vi "SendDrivingCAN.vi"(11 "CANTXQueueIn":T1) -> (3 "CANTXQueueOut":T1)   [LabVIEW 2015]
uses:
  CAN/TX Library/CAN Message Queue.ctl
  CAN/TX Library/CAN Message.ctl
  <vilib>/RioEmbeddedCAN/RioEmbeddedCAN.llb/CANFrameControl.ctl
  Global Data.vi
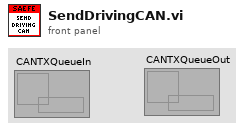
[diagram p1: front panel]
types:
  T1 = typedef "CAN Message Queue.ctl" = refnum<k33>
  T2 = typedef "CANFrameControl.ctl" = cluster{"identifier":u32, "extended?":bool, "type":u8, "payload":u8[]}
  T3 = typedef "Lap Statistics.ctl" = cluster{"rBrakeBalLast":dbl}
  T4 = typedef "MC Temp 2.ctl" = cluster{"TMCControlBoard":dbl, "TMCRTD1":dbl, "TMCRTD2":dbl, "TMCRTD3":dbl}
  T5 = typedef "BMS Telemetry.ctl" = cluster{"bBMSIgnition":bool, "bBMSChargerMains":bool, "bBMSFastCharge":bool, "bBMSChargerEnabled":bool, "eBMSCarState":enum16{"Off", "On, Not Charging", "Charging", "Charging Finished", "Charging Error"}, "eBMSChargingState":enum16{"Disconnected", "Pre-charging", "Main Charging", "Balancing", "Charging Finished OK", "Charging Error"}, "tBMSChargeStage":u16, "eBMSLastChargeError":enum16{"No Error", "No Cell Communication", "No Cell Communication - Non CAN Charger", "Maximum charging stage duration expired", "Cell Communication Lost during Charge", "Cannot set balancing voltage", "Cell temps too high", "No Comms so can't determine temp", "# of Cells Mismatch", "Cells Overvoltage", "Cell Protection Event occured."}, "NBMSNumCells":u8, "bBMSUnderVProtection":bool, "bBMSOverVProtection":bool, "bBMSOverTProtection":bool, "bBMSLeakageProtection":bool, "bBMSNoCellCommsError":bool, "bBMSLowVReduction":bool, "bBMSHighTReduction":bool, "VCellMin":dbl, "VCellMax":dbl, "VCellMean":dbl, "VTotal":dbl, "TCellMin":dbl, "TCellMax":dbl, "TCellMean":dbl, "VCells":cluster{"[51]":dbl, "[53]":dbl, "[54]":dbl, "[55]":dbl, "[56]":dbl, "[57]":dbl, "[58]":dbl, "[59]":dbl, "[60]":dbl, "[61]":dbl, "[62]":dbl, "[63]":dbl, "[64]":dbl, "[65]":dbl, "[66]":dbl, "[67]":dbl, "[34]":dbl, "[35]":dbl, "[36]":dbl, "[37]":dbl, "[38]":dbl, "[39]":dbl, "[40]":dbl, "[41]":dbl, "[42]":dbl, "[43]":dbl, "[44]":dbl, "[45]":dbl, "[46]":dbl, "[47]":dbl, "[48]":dbl, "[49]":dbl, "[50]":dbl, "[17]":dbl, "[18]":dbl, "[19]":dbl, "[20]":dbl, "[21]":dbl, "[22]":dbl, "[23]":dbl, "[24]":dbl, "[25]":dbl, "[26]":dbl, "[27]":dbl, "[28]":dbl, "[29]":dbl, "[30]":dbl, "[31]":dbl, "[32]":dbl, "[33]":dbl, "[0]":dbl, "[1]":dbl, "[2]":dbl, "[3]":dbl, "[4]":dbl, "[5]":dbl, "[6]":dbl, "[7]":dbl, "[8]":dbl, "[9]":dbl, "[10]":dbl, "[11]":dbl, "[12]":dbl, "[13]":dbl, "[14]":dbl, "[15]":dbl, "[16]":dbl, "[52] 2":dbl}, "TBMSCells":cluster{"[55]":dbl, "[56]":dbl, "[57]":dbl, "[58]":dbl, "[59]":dbl, "[60]":dbl, "[61]":dbl, "[62]":dbl, "[63]":dbl, "[64]":dbl, "[65]":dbl, "[66]":dbl, "[67]":dbl, "[68]":dbl, "[69]":dbl, "[70]":dbl, "[17]":dbl, "[38]":dbl, "[39]":dbl, "[40]":dbl, "[41]":dbl, "[42]":dbl, "[43]":dbl, "[44]":dbl, "[45]":dbl, "[46]":dbl, "[47]":dbl, "[48]":dbl, "[49]":dbl, "[50]":dbl, "[51]":dbl, "[52]":dbl, "[53]":dbl, "[54]":dbl, "[21]":dbl, "[22]":dbl, "[23]":dbl, "[24]":dbl, "[25]":dbl, "[26]":dbl, "[27]":dbl, "[28]":dbl, "[29]":dbl, "[30]":dbl, "[31]":dbl, "[32]":dbl, "[33]":dbl, "[34]":dbl, "[35]":dbl, "[36]":dbl, "[37]":dbl, "[0]":dbl, "[1]":dbl, "[2]":dbl, "[3]":dbl, "[4]":dbl, "[5]":dbl, "[6]":dbl, "[7]":dbl, "[8]":dbl, "[9]":dbl, "[10]":dbl, "[11]":dbl, "[12]":dbl, "[13]":dbl, "[14]":dbl, "[15]":dbl, "[16]":dbl}, "bChargerConnected":bool, "VChargerSetpoint":dbl, "IChargerSetpoint":dbl, "VChargerActual":dbl, "IChargerActual":dbl, "BCells":cluster{"[51]":dbl, "[52]":dbl, "[53]":dbl, "[54]":dbl, "[55]":dbl, "[56]":dbl, "[57]":dbl, "[58]":dbl, "[59]":dbl, "[60]":dbl, "[61]":dbl, "[62]":dbl, "[63]":dbl, "[64]":dbl, "[65]":dbl, "[66]":dbl, "[67]":dbl, "[34]":dbl, "[35]":dbl, "[36]":dbl, "[37]":dbl, "[38]":dbl, "[39]":dbl, "[40]":dbl, "[41]":dbl, "[42]":dbl, "[43]":dbl, "[44]":dbl, "[45]":dbl, "[46]":dbl, "[47]":dbl, "[48]":dbl, "[49]":dbl, "[50]":dbl, "[17]":dbl, "[18]":dbl, "[19]":dbl, "[20]":dbl, "[21]":dbl, "[22]":dbl, "[23]":dbl, "[24]":dbl, "[25]":dbl, "[26]":dbl, "[27]":dbl, "[28]":dbl, "[29]":dbl, "[30]":dbl, "[31]":dbl, "[32]":dbl, "[33]":dbl, "[0]":dbl, "[1]":dbl, "[2]":dbl, "[3]":dbl, "[4]":dbl, "[5]":dbl, "[6]":dbl, "[7]":dbl, "[8]":dbl, "[9]":dbl, "[10]":dbl, "[11]":dbl, "[12]":dbl, "[13]":dbl, "[14]":dbl, "[15]":dbl, "[16]":dbl}, "bNewVCellMinSample":bool, "Battery Temp":cluster{"[0]":dbl, "[1]":dbl, "[2]":dbl, "[3]":dbl, "[4]":dbl, "[5]":dbl, "[6]":dbl, "[7]":dbl, "[8]":dbl, "[9]":dbl, "[10]":dbl, "[11]":dbl, "[12]":dbl, "[13]":dbl, "[14]":dbl, "[15]":dbl, "[16]":dbl, "[17]":dbl, "[18]":dbl, "[19]":dbl, "[20]":dbl, "[21]":dbl, "[22]":dbl, "[23]":dbl, "[24]":dbl, "[25]":dbl, "[26]":dbl, "[27]":dbl, "[28]":dbl, "[29]":dbl, "[30]":dbl, "[31]":dbl, "[32]":dbl, "[33]":dbl, "[34]":dbl, "[35]":dbl, "[36]":dbl, "[37]":dbl, "[38]":dbl, "[39]":dbl, "[40]":dbl, "[41]":dbl, "[42]":dbl, "[43]":dbl, "[44]":dbl, "[45]":dbl, "[46]":dbl, "[47]":dbl, "[48]":dbl, "[49]":dbl, "[50]":dbl, "[51]":dbl, "[52]":dbl, "[53]":dbl, "[54]":dbl, "[55]":dbl, "[56]":dbl, "[57]":dbl, "[58]":dbl, "[59]":dbl, "[60]":dbl, "[61]":dbl, "[62]":dbl, "[63]":dbl, "[64]":dbl, "[65]":dbl, "[66]":dbl, "[67]":dbl, "[68]":dbl, "[69]":dbl, "[71]":dbl, "[70]":dbl, "[0] 2":dbl, "[1] 2":dbl, "[2] 2":dbl, "[3] 2":dbl, "[4] 2":dbl, "[5] 2":dbl, "[6] 2":dbl, "[7] 2":dbl, "[8] 2":dbl, "[9] 2":dbl, "[10] 2":dbl, "[11] 2":dbl, "[12] 2":dbl, "[13] 2":dbl, "[14] 2":dbl, "[15] 2":dbl, "[16] 2":dbl, "[17] 2":dbl, "[18] 2":dbl, "[19] 2":dbl, "[20] 2":dbl, "[21] 2":dbl, "[22] 2":dbl, "[23] 2":dbl, "[24] 2":dbl, "[25] 2":dbl, "[26] 2":dbl, "[27] 2":dbl, "[28] 2":dbl, "[29] 2":dbl, "[30] 2":dbl, "[31] 2":dbl, "[32] 2":dbl, "[33] 2":dbl, "[34] 2":dbl, "[35] 2":dbl, "[36] 2":dbl, "[37] 2":dbl, "[38] 2":dbl, "[39] 2":dbl, "[40] 2":dbl, "[41] 2":dbl, "[42] 2":dbl, "[43] 2":dbl, "[44] 2":dbl, "[45] 2":dbl, "[46] 2":dbl, "[47] 2":dbl, "[48] 2":dbl, "[49] 2":dbl, "[50] 2":dbl, "[51] 2":dbl, "[52] 3":dbl, "[53] 2":dbl, "[54] 2":dbl, "[55] 2":dbl, "[56] 2":dbl, "[57] 2":dbl, "[58] 2":dbl, "[59] 2":dbl, "[60] 2":dbl, "[61] 2":dbl, "[62] 2":dbl, "[63] 2":dbl, "[64] 2":dbl, "[65] 2":dbl, "[66] 2":dbl, "[67] 2":dbl, "[68]2":dbl, "[69]2":dbl, "[70]2":dbl, "[71]2":dbl, "[0] 3":dbl, "[1] 3":dbl, "[2] 3":dbl, "[3] 3":dbl, "[4] 3":dbl, "[5] 3":dbl, "[6] 3":dbl, "[7] 3":dbl, "[8] 3":dbl, "[9] 3":dbl, "[10] 3":dbl, "[11] 3":dbl, "[12] 3":dbl, "[13] 3":dbl, "[14] 3":dbl, "[15] 3":dbl, "[16] 3":dbl, "[17] 3":dbl, "[18] 3":dbl, "[19] 3":dbl, "[20] 3":dbl, "[21] 3":dbl, "[22] 3":dbl, "[23] 3":dbl, "[24] 3":dbl, "[25] 3":dbl, "[26] 3":dbl, "[27] 3":dbl, "[28] 3":dbl, "[29] 3":dbl, "[30] 3":dbl, "[31] 3":dbl, "[32] 3":dbl, "[33] 3":dbl, "[34] 3":dbl, "[35] 3":dbl, "[36] 3":dbl, "[37] 3":dbl, "[38] 3":dbl, "[39] 3":dbl, "[40] 3":dbl, "[41] 3":dbl, "[42] 3":dbl, "[43] 3":dbl, "[44] 3":dbl, "[45] 3":dbl, "[46] 3":dbl, "[47] 3":dbl, "[48] 3":dbl, "[49] 3":dbl, "[50] 3":dbl, "[51] 3":dbl, "[52] 4":dbl, "[53] 3":dbl, "[54] 3":dbl, "[55] 3":dbl, "[56] 3":dbl, "[57] 3":dbl, "[58] 3":dbl, "[59] 3":dbl, "[60] 3":dbl, "[61] 3":dbl, "[62] 3":dbl, "[63] 3":dbl, "[64] 3":dbl, "[65] 3":dbl, "[66] 3":dbl, "[67] 3":dbl, "[68]3":dbl, "[69]3":dbl, "[70]3":dbl, "[71]3":dbl, "[4] 4":dbl, "[5] 4":dbl, "[6] 4":dbl, "[7] 4":dbl, "[8] 4":dbl, "[9] 4":dbl, "[10] 4":dbl, "[11] 4":dbl, "[12] 4":dbl, "[13] 4":dbl, "[14] 4":dbl, "[15] 4":dbl, "[16] 4":dbl, "[17] 4":dbl, "[18] 4":dbl, "[19] 4":dbl, "[20] 4":dbl, "[21] 4":dbl, "[22] 4":dbl, "[23] 4":dbl, "[24] 4":dbl, "[25] 4":dbl, "[26] 4":dbl, "[27] 4":dbl, "[28] 4":dbl, "[29] 4":dbl, "[30] 4":dbl, "[31] 4":dbl, "[32] 4":dbl, "[33] 4":dbl, "[17] 9":dbl, "[0] 9":dbl, "[51] 8":dbl, "[34] 8":dbl, "[17] 8":dbl, "[0] 8":dbl, "[34] 4":dbl, "[35] 4":dbl, "[36] 4":dbl, "[37] 4":dbl, "[38] 4":dbl, "[39] 4":dbl, "[40] 4":dbl, "[41] 4":dbl, "[42] 4":dbl, "[43] 4":dbl, "[44] 4":dbl, "[45] 4":dbl, "[46] 4":dbl, "[47] 4":dbl, "[48] 4":dbl, "[49] 4":dbl, "[50] 4":dbl, "[34] 9":dbl, "[51] 4":dbl, "[52] 5":dbl, "[53] 4":dbl, "[54] 4":dbl, "[55] 4":dbl, "[56] 4":dbl, "[57] 4":dbl, "[58] 4":dbl, "[59] 4":dbl, "[60] 4":dbl, "[61] 4":dbl, "[62] 4":dbl, "[63] 4":dbl, "[64] 4":dbl, "[65] 4":dbl, "[66] 4":dbl, "[67] 4":dbl, "[51] 9":dbl}, "TBMSMax":dbl, "TBMSMin":dbl, "TBMSMean":dbl}
  T6 = typedef "MC Temp 1.ctl" = cluster{"TMCModuleA":dbl, "TMCModuleB":dbl, "TMCModuleC":dbl, "TMCGateDriver":dbl}
  T7 = typedef "MC Temp 3.ctl" = cluster{"TMCRTD4":dbl, "TMCRTD5":dbl, "TMotor":dbl, "MTorqueShudder":dbl}
  T8 = typedef "FPGA Telemetry.ctl" = cluster{"CPU Load":cluster{"Total (%)":dbl, "Time Critical (%)":dbl, "Timed Structures (%)":dbl, "High (%)":dbl, "Above Normal (%)":dbl, "Normal (%)":dbl, "Background (%)":dbl, "Idle (%)":dbl, "ISR (%)":dbl}, "SVehicleStatus":cluster{"BMS Status":T9, "MC Status":T9, "Shutdown Status":T9, "sbRIO Status":T9, "Vehicle Status":T9, "Shutdown State":enum16{"NI.SC.Initial", "NI.SC.History", "NI.SC.ShallowHistory", "NI.SC.Terminal", "Coolant Pump Started/AIR's On", "AIRs On", "Precharge", "TSMS Off"}, "AIR Status":T12, "Remote Return to Pits":bool, "Reason for Shutdown":T13, "MC State Machine Status":enum16{"NI.SC.Initial", "NI.SC.History", "NI.SC.ShallowHistory", "NI.SC.Terminal", "Broadcast Diag", "Let Current Drop then Disable AIR's", "Enabled", "Disabled"}}, "iPhone HF Data":cluster{"gXiPhone":dbl, "gYiPhone":dbl, "gZiPhone":dbl, "nYawXiPhone":dbl, "nYawYiPhone":dbl, "nYawZiPhone":dbl}, "iPhone LF Data":cluster{"nLatiPhone":dbl, "nLongiPhone":dbl, "nGPSiPhone":dbl}, "stop":bool, "VSupplyOffset":fxp<+,12,4>, "VsbRIOSupply":fxp<+/-,25,6>, "bFPGALED":bool, "TSBRIO":fxp<+/-,33,17>, "rTPS2Unscaled":fxp<+/-,16,1>, "rTPS1Unscaled":fxp<+/-,16,1>, "bTPSConsistent":bool, "bTPSInRange":bool, "rThrottle":fxp<+/-,33,22>, "VTPS2":fxp<+/-,24,5>, "rTPS2":fxp<+/-,31,22>, "VTPS1":fxp<+/-,24,5>, "rTPS1":fxp<+/-,31,22>, "rTPS2Max":fxp<+,16,4>, "rTPS2Min":fxp<+,16,4>, "rTPS1Max":fxp<+,16,4>, "rTPS1Min":fxp<+,16,4>, "bCoolantPumpEnable":bool, "bRTDSEnable":bool, "bTSMSInStatus":bool, "bPosAIREnable":bool, "bBMSOK":bool, "bIMDOK":bool, "bBSPDOK":bool, "bSBRIOOK2":bool, "bSBRIOOK1":bool, "bTSMSOutStatus":bool, "eGreenDash":T14, "eYellowDash":T14, "eRedDash":T14, "bMotorControllerEnable":bool, "tCurrentLap":u32, "bNewLap":bool, "tLastLap":u32, "tLapMin":u32, "V5VSupply":fxp<+/-,24,5>, "bWheelRL":bool, "bWheelRR":bool, "bWheelFR":bool, "bWheelFL":bool, "VBrakePressureR":fxp<+/-,24,5>, "VBrakePressureF":fxp<+/-,24,5>, "bWheelRRStopped":bool, "bWheelRLStopped":bool, "bWheelFRStopped":bool, "bWheelFLStopped":bool, "tWheelRLPeriod":u32, "tWheelRRPeriod":u32, "tWheelFRPeriod":u32, "tWheelFLPeriod":u32, "bBrakeLight":bool, "VShockRR":fxp<+/-,24,5>, "VShockRL":fxp<+/-,24,5>, "VShockFR":fxp<+/-,24,5>, "VShockFL":fxp<+/-,24,5>, "IHighCurrent":fxp<+/-,24,15>, "ILowCurrent":fxp<+/-,24,15>, "pBrakeR":fxp<+,26,13>, "pBrakeF":fxp<+,26,13>, "bHighCurrentOK":bool, "bLowCurrentOK":bool, "bBrakeROK":bool, "bBrakeFOK":bool, "VSteerWheelMiddle":fxp<+/-,26,5>, "aSteerWheel":fxp<+/-,31,13>, "nWheelFL":fxp<+/-,32,16>, "nWheelFR":fxp<+/-,32,16>, "nWheelRL":fxp<+/-,32,16>, "nWheelRR":fxp<+/-,32,16>, "ADXL345 Output":T15, "Tire Diameter(m)":fxp<+,16,1>, "vWheelRR":fxp<+/-,32,18>, "vWheelRL":fxp<+/-,32,18>, "vWheelFR":fxp<+/-,32,18>, "vWheelFL":fxp<+/-,32,18>, "vWheelLowest":fxp<+/-,32,18>, "vWheelHighest":fxp<+/-,32,18>, "bAccel":bool, "vAxleF":fxp<+/-,33,19>, "vCar":fxp<+/-,33,19>, "sLap":fxp<+,32,12>, "rSlipRL":fxp<+/-,12,1>, "rSlipRR":fxp<+/-,12,1>, "rSlipFL":fxp<+/-,12,1>, "rSlipFR":fxp<+/-,12,1>, "NLap":u8, "tLapReference":u32, "tFastestLap":u32, "MTorqueRequest":dbl, "RS232 Error Out":cluster{"status":bool, "code":i32}}
  T9 = typedef "Subsystem Status.ctl" = cluster{"eStatusSeverity":T10, "NValue":sgl, "CMessage":T11, "bNotOK":bool}
  T10 = typedef "Subsystem Status Severity.ctl" = enum16{"Okay", "Short Warning", "Long Warning", "Return to Pits", "Error", "Danger"}
  T11 = typedef "Subsystem Status Message.ctl" = enum16{"ControllerTemperature", "MotorTemperature", "BatteryTemperature", "BatteryLowVoltage", "LVBattery", "sbRIOTemperature", "Precharge", "BSPD", "IMD", "RemoteReturnToPits", "EStopInterrupted", "NoCellComms", "MCOverSpeed", "MCOverCurrent", "MCOverVoltage", "MCInverterOverTemp", "MCDirectionCommand", "MCInverterTimeout", "MCDesatFault", "MCHWOverCurrent", "MCUnderVoltage", "MCCommandMessageLost", "MotorOverTemp", "MCModAOverTemp", "MCModBOverTemp", "MCModCOverTemp", "MCPCBOverTemp", "MCGateDrv1OverTemp", "MCDateDrv2OverTemp", "MCCurrentSensorFault", "MCResolverNotConnected", "ShutdownLatchTripped", "UnknownBMS", "RemoteEmergency"}
  T12 = typedef "AIR Status.ctl" = enum16{"Off", "Precharge", "On"}
  T13 = typedef "Reason for Shutdown.ctl" = enum16{"None", "BMS", "Shutdown", "sbRIO", "MC", "Remote"}
  T14 = typedef "Dash LED Status.ctl" = enum16{"Off", "Flashing", "On"}
  T15 = typedef "ADXL345 Output.ctl" = cluster{"X":fxp<+/-,14,4>, "Y":fxp<+/-,14,4>, "Z":fxp<+/-,14,4>}
  T16 = typedef "Shutdown State Machine.lvsc/State.ctl" = enum16{"NI.SC.Initial", "NI.SC.History", "NI.SC.ShallowHistory", "NI.SC.Terminal", "Coolant Pump Started/AIR's On", "AIRs On", "Precharge", "TSMS Off"}
  T17 = typedef "MC State Machine.lvsc/State.ctl" = enum16{"NI.SC.Initial", "NI.SC.History", "NI.SC.ShallowHistory", "NI.SC.Terminal", "Broadcast Diag", "Let Current Drop then Disable AIR's", "Enabled", "Disabled"}
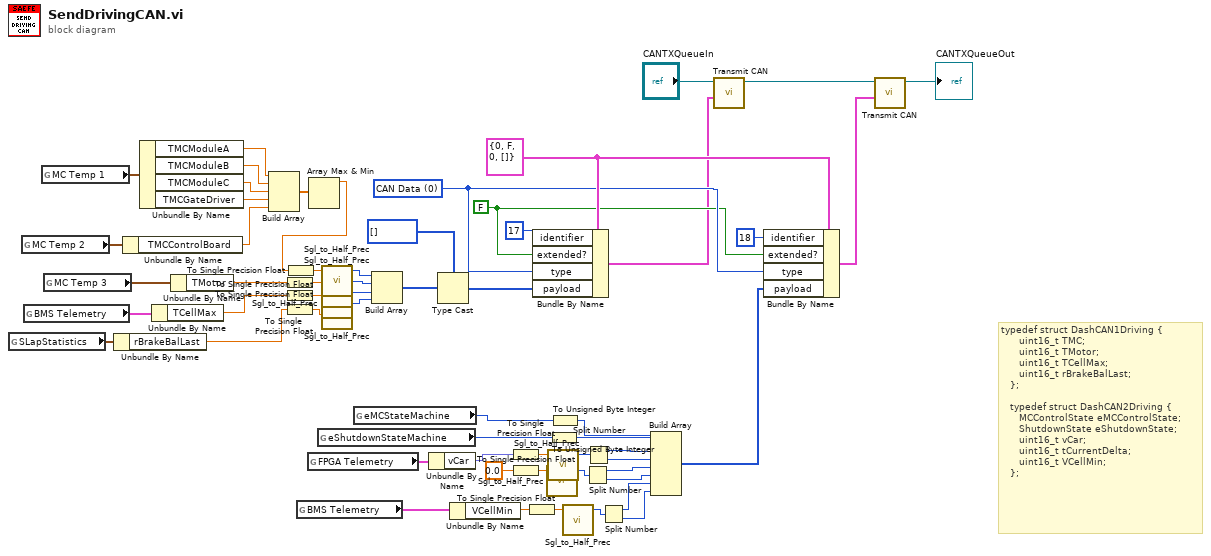
[diagram p0: block diagram]
diagram:
  w55 = u8 0 items=["CAN Data", "CAN Remote"] ("type")
  w57 = T2 {"identifier"=0, "extended?"=FALSE, "type"=0, "payload"=[]} ("CAN frame")
  w54 = FALSE ("extended?")
  # "typedef struct DashCAN1Driving {\n      uint16_t TMC;\n      uint16_t TMotor;\n      uint16_t TCellMax;\n      uint16_t rBrakeBalLast;\n   };\n\n   typedef struct DashCAN2Driving {\n      MCControlState eMCControlState;\n      ShutdownState eShutdownState;\n      uint16_t vCar;\n      uint16_t tCurrentDelta;\n      uint16_t VCellMin;\n   };"
  n1 = global read "Global Data.vi" "SLapStatistics"() -> (w15:T3)
  n2 = global read "Global Data.vi" "MC Temp 2"() -> (w42:T4)
  n3 = global read "Global Data.vi" "BMS Telemetry"() -> (w33:T5)
  n4 = global read "Global Data.vi" "MC Temp 1"() -> (w43:T6)
  n5 = global read "Global Data.vi" "MC Temp 3"() -> (w46:T7)
  n6 = Unbundle By Name(w15) -> ("rBrakeBalLast"=w13:dbl)
  n7 = Unbundle By Name(w42) -> ("TMCControlBoard"=w37:dbl)
  n8 = Unbundle By Name(w43) -> ("TMCModuleA"=w41:dbl, "TMCModuleB"=w40:dbl, "TMCModuleC"=w39:dbl, "TMCGateDriver"=w38:dbl)
  n9 = Unbundle By Name(w33) -> ("TCellMax"=w31:dbl)
  n10 = Unbundle By Name(w46) -> ("TMotor"=w45:dbl)
  n11 = Build Array(w41, w40, w39, w38, w37) -> (w36:dbl[])
  n12 = To Single Precision Float(number=w45) -> (single precision float=w44:sgl)
  n13 = To Single Precision Float(number=w31) -> (single precision float=w32:sgl)
  n14 = To Single Precision Float(number=w13) -> (single precision float=w14:sgl)
  n15 = global read "Global Data.vi" "BMS Telemetry"() -> (w11:T5)
  n16 = global read "Global Data.vi" "FPGA Telemetry"() -> (w17:T8)
  n17 = Array Max & Min(array=w36) -> (max value=w34:dbl)  [unwired: 3 out]
  n18 = To Single Precision Float(number=w34) -> (single precision float=w35:sgl)
  n19 = global read "Global Data.vi" "eShutdownStateMachine"() -> (w18:T16)
  n20 = call "Sgl_to_Half_Prec.vi"("SGL"=w35) -> ("Half Precision Floating Point"=w50:u16)  [unwired: 4 in]
  n21 = call "Sgl_to_Half_Prec.vi"("SGL"=w44) -> ("Half Precision Floating Point"=w49:u16)  [unwired: 4 in]
  n22 = call "Sgl_to_Half_Prec.vi"("SGL"=w32) -> ("Half Precision Floating Point"=w48:u16)  [unwired: 4 in]
  n23 = call "Sgl_to_Half_Prec.vi"("SGL"=w14) -> ("Half Precision Floating Point"=w47:u16)  [unwired: 4 in]
  n24 = global read "Global Data.vi" "eMCStateMachine"() -> (w19:T17)
  n25 = Build Array(w50, w49, w48, w47) -> (w51:u16[])
  n26 = Unbundle By Name(w17) -> ("vCar"=w16:fxp<+/-,33,19>)
  n27 = Type Cast(type=u8[] [], x=w51) -> (*(type *) &x=w53:u8[])
  n28 = Unbundle By Name(w11) -> ("VCellMin"=w8:dbl)
  n29 = To Single Precision Float(number=w16) -> (single precision float=w30:sgl)
  n30 = To Single Precision Float(number=sgl 0.0) -> (single precision float=w29:sgl)
  n31 = To Single Precision Float(number=w8) -> (single precision float=w10:sgl)
  n32 = Bundle By Name(cluster=w57, "identifier"=u32 17, "extended?"=w54, "type"=w55, "payload"=w53) -> (w2:T2)
  n33 = call "Sgl_to_Half_Prec.vi"("SGL"=w29) -> ("Half Precision Floating Point"=w28:u16)  [unwired: 4 in]
  n34 = call "Sgl_to_Half_Prec.vi"("SGL"=w30) -> ("Half Precision Floating Point"=w27:u16)  [unwired: 4 in]
  n35 = To Unsigned Byte Integer(number=w18) -> (unsigned 8bit integer=w25:u8)
  n36 = To Unsigned Byte Integer(number=w19) -> (unsigned 8bit integer=w26:u8)
  n37 = call "Sgl_to_Half_Prec.vi"("SGL"=w10) -> ("Half Precision Floating Point"=w9:u16)  [unwired: 4 in]
  n38 = Split Number(x=w28) -> (hi(x)=w22:u8, lo(x)=w21:u8)
  n39 = Split Number(x=w27) -> (hi(x)=w24:u8, lo(x)=w23:u8)
  n40 = Split Number(x=w9) -> (hi(x)=w7:u8, lo(x)=w6:u8)
  n41 = Build Array(w26, w25, w24, w23, w22, w21, w7, w6) -> (w20:u8[])
  n42 = call "Transmit CAN.vi"("CAN Queue"="CANTXQueueIn", "CAN frame"=w2) -> ("CAN Queue Out"=w4:T1)  [unwired: 8 in]
  n43 = Bundle By Name(cluster=w57, "identifier"=u32 18, "extended?"=w54, "type"=w55, "payload"=w20) -> (w1:T2)
  n44 = call "Transmit CAN.vi"("CAN Queue"=w4, "CAN frame"=w1) -> ("CAN Queue Out"=→"CANTXQueueOut":T1)  [unwired: 8 in]
